vi "Perform Work.vi"(4 "Controller name":string, 6 "Last request":bool, 7 "Update period":dbl, 8 "error in (no error)":errorcluster, 9 "Initialize":bool, 11 "Measure Controller in":refnum<class "Process Controller.lvclass">) -> (0 "error out":errorcluster, 3 "Measure Controller out":refnum<class "Process Controller.lvclass">)   [LabVIEW 2021, in "Process Controller.lvclass"]
uses:
  Process Controller.lvclass
  Process Controller.lvclass/Process Controller.ctl
  Read Active measurements names.vi
  Measurements/Response Synchronizer/Response Synchronizer.lvclass
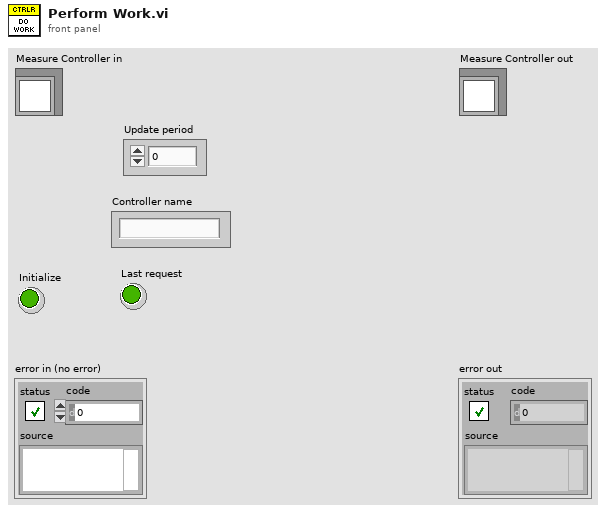
[diagram p1: front panel]
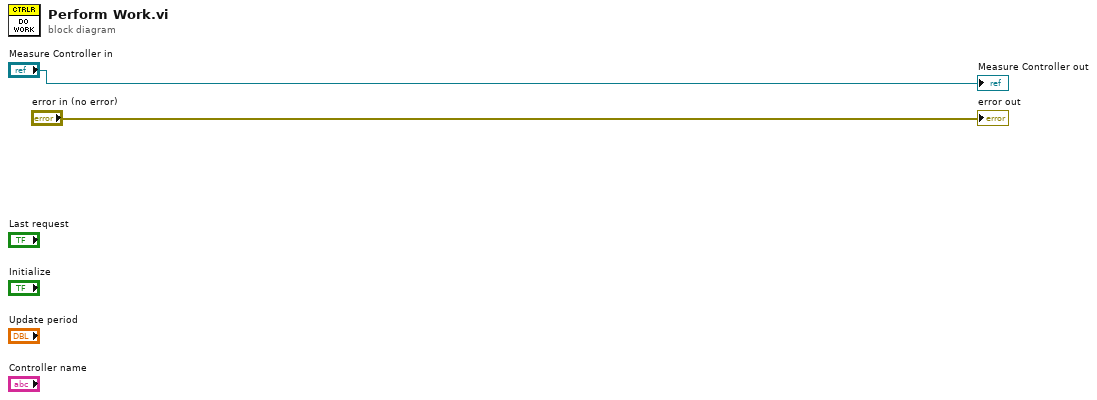
[diagram p0: block diagram]
diagram:
  "error out" <- "error in (no error)"
  "Measure Controller out" <- "Measure Controller in"
